vi "DAQmx Create Channel (AI-Strain-Strain Gage).vi"(0 "task in":refnum<k21>, 1 "maximum value":dbl=0.001 format="%0.7f", 2 "minimum value":dbl=-0.001 format="%0.7f", 5 "physical channels":tag, 7 "name to assign":string, 9 "units":i32(ring)=10299 items=["Strain"=10299, "From Custom Scale"=10065], 11 "error in":errorcluster, 12 "custom scale name":tag, 13 "bridge information":T1={"strain configuration"=10183, "lead wire resistance"=0.0, "initial bridge voltage"=0.0, "voltage excitation source"=10200, "voltage excitation value"=2.5} {"initial bridge voltage" format="%0.2f"; "voltage excitation source" items=["Internal"=10200, "External"=10167, "None"=10230]; "voltage excitation value" format="%0.2f"; "lead wire resistance" format="%0.2f"; "strain configuration" items=["Full Bridge I"=10183, "Full Bridge II"=10184, "Full Bridge III"=10185, "Half Bridge I"=10188, "Half Bridge II"=10189, "Quarter Bridge I"=10271, "Quarter Bridge II"=10272]}, 14 "strain gage information":T2={"gage factor"=2.0, "nominal gage resistance"=350.0, "poisson ratio"=0.3} {"poisson ratio" format="%0.2f"; "nominal gage resistance" format="%0.2f"; "gage factor" format="%0.2f"}) -> (4 "task out":refnum<k21>, 15 "error out":errorcluster)   [LabVIEW 2020]
doc: "Creates channel(s) to measure strain."
uses:
  nilvaiu.dll
panel:
  # "input limits"
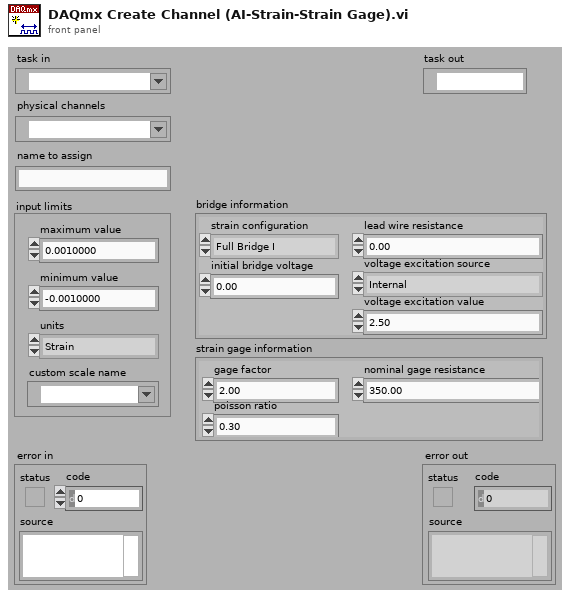
[diagram p1: front panel]
types:
  T1 = cluster{"strain configuration":i32, "lead wire resistance":dbl, "initial bridge voltage":dbl, "voltage excitation source":i32, "voltage excitation value":dbl}
  T2 = cluster{"gage factor":dbl, "nominal gage resistance":dbl, "poisson ratio":dbl}
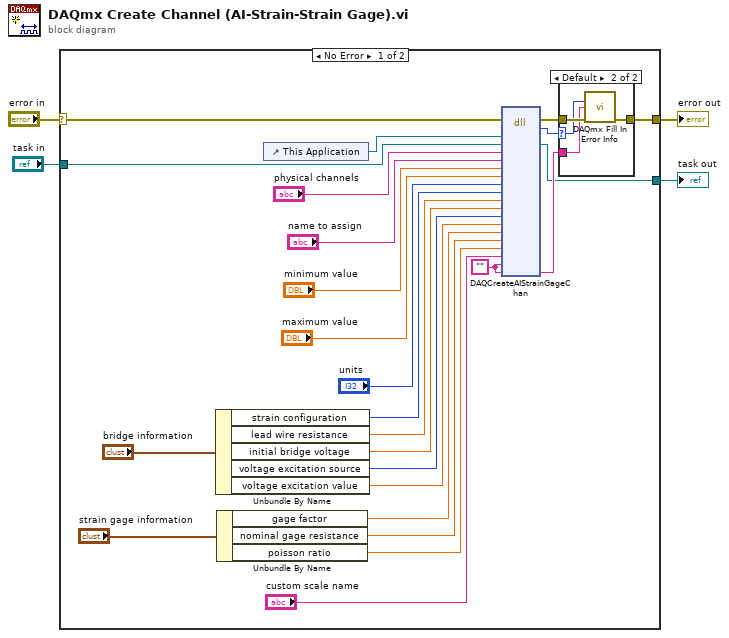
[diagram p0: block diagram]
diagram:
  n1 = case shown="No Error" "error in" {
    selector: "error in" -> [w22 w35]
    tunnel: [w7 w35] -> w4
    tunnel: "task in" -> [w26 w36]
    tunnel: [w9 w36] -> w1
    frame No Error {
      w5 = ""
      n2 = Unbundle By Name("bridge information") -> ("strain configuration"=w18:i32, "lead wire resistance"=w17:dbl, "initial bridge voltage"=w16:dbl, "voltage excitation source"=w15:i32, "voltage excitation value"=w14:dbl)
      n3 = Unbundle By Name("strain gage information") -> ("gage factor"=w13:dbl, "nominal gage resistance"=w12:dbl, "poisson ratio"=w11:dbl)
      n4 = control-ref of="This Application"() -> (w27:refnum<vi>)
      n5 = dll-call lib="nilvaiu.*" fn="DAQCreateAIStrainGageChan"(error in=w22, "lvAppRef"=w27, "refObjPtr"=w26, "physicalChannelName"="physical channels", "channelNameIn"="name to assign", "minVal"="minimum value", "maxVal"="maximum value", "units"="units", "strainConfig"=w18, "leadWireResist"=w17, "initialBridgeVoltage"=w16, "excitSource"=w15, "excitValue"=w14, "gageFactor"=w13, "nominalGageResist"=w12, "poissonRatio"=w11, "customScaleName"="custom scale name", "channelNamesOut"=w5, "extendedErrorInfo"=w5) -> (error out=w8:errorcluster, "return type"=w6:i32, "refObjPtr"=w9:refnum<k21>, "extendedErrorInfo"=w10:string)  [unwired: 18 in, 1 out]
      n6 = case shown="Default" w6 {
        selector: w6 -> [_ w32]
        tunnel: w8 -> [w30 w34]
        tunnel: [w30 w33] -> w7
        tunnel: w10 -> [_ w31]
        frame 0 {
        }
        frame Default {
          n7 = call "DAQmx Fill In Error Info.vi"("status code"=w32, "extended error info"=w31, "error in"=w34) -> ("error out"=w33:errorcluster)  [unwired: 1 in, 11 out]
        }
      }
    }
    frame Error {
    }
  }
  "error out" <- w4
  "task out" <- w1
